vi "REPORT_AUDIT_get_data_results.vi"(6 "executed_SQL_statement_in":string, 8 "error_in":errorcluster, 11 "SQL_result":variant) -> (0 "error_out":errorcluster, 4 "executed_SQL_statement_out":string)   [LabVIEW 2020]
uses:
  FGV/SQL_connection/FGV_CLIENT_SQL_connection.ctl
  FGV/REPORTS_records_display/FGV_REPORTS_records_display.ctl
  _misc/AULocalize/SubVIs/Get Localized Phrase Compact Interface 0D.vi
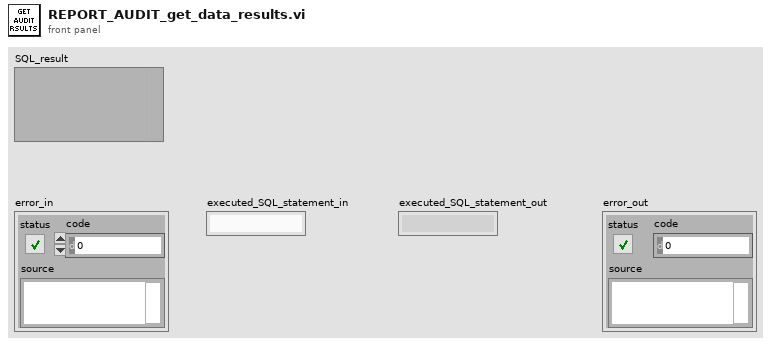
[diagram p1: front panel]
types:
  T1 = typedef "FGV_REPORTS_records_display.ctl" = enum16{"initialize", "GEAR_set_serial", "GEAR_set_header", "GEAR_set_operations", "GEAR_set_results", "GEAR_set_batches", "GEAR_get_serial", "GEAR_get_operation_IDs", "GEAR_toggle_results", "GEAR_show_all_results", "GEAR_hide_all_results", "GEAR_display", "GEAR_filter", "GEAR_restore", "GEAR_clear", "GEAR_get_all_info", "DATES_set_dates", "DATES_set_gears", "DATES_display", "DATES_filter", "DATES_first_page", "DATES_previous_page", "DATES_next_page", "DATES_last_page", "DATES_restore", "DATES_clear", "DATES_get_all_info", "PBATCH_set_batch_no", "PBATCH_set_gears", "PBATCH_display", "PBATCH_filter", "PBATCH_first_page", "PBATCH_previous_page", "PBATCH_next_page", "PBATCH_last_page", "PBATCH_restore", "PBATCH_clear", "PBATCH_get_all_info", "OPRTN_set_OP", "OPRTN_set_dates", "OPRTN_set_gears", "OPRTN_set_hidden_columns", "OPRTN_display", "OPRTN_filter", "OPRTN_filter_no_page_reset", "OPRTN_first_page", "OPRTN_previous_page", "OPRTN_next_page", "OPRTN_last_page", "OPRTN_restore", "OPRTN_clear", "OPRTN_get_all_info", "CFG_set_type", "CFG_set_dates", "CFG_set_records", "CFG_display", "CFG_filter", "CFG_first_page", "CFG_previous_page", "CFG_next_page", "CFG_last_page", "CFG_restore", "CFG_clear", "CFG_get_all_info", "AUDIT_set_dates", "AUDIT_set_records", "AUDIT_display", "AUDIT_filter", "AUDIT_first_page", "AUDIT_previous_page", "AUDIT_next_page", "AUDIT_last_page", "AUDIT_restore", "AUDIT_clear", "AUDIT_set_results", "AUDIT_get_all_info", "AUDIT_toggle_results", "AUDIT_show_all_results", "AUDIT_hide_all_results", "OKNOK_set_dates", "OKNOK_set_records", "OKNOK_display", "OKNOK_restore", "OKNOK_clear", "OKNOK_get_all_info", "REWORKS_set_dates", "REWORKS_set_from_to", "REWORKS_set_records", "REWORKS_display", "REWORKS_filter", "REWORKS_first_page", "REWORKS_previous_page", "REWORKS_next_page", "REWORKS_last_page", "REWORKS_restore", "REWORKS_clear", "REWORKS_get_all_info", "PACE_set_dates", "PACE_set_limits", "PACE_set_records", "PACE_display", "PACE_restore", "PACE_clear", "PACE_get_all_info", "CBATCH_set_code", "CBATCH_set_records", "CBATCH_display", "CBATCH_filter", "CBATCH_first_page", "CBATCH_previous_page", "CBATCH_next_page", "CBATCH_last_page", "CBATCH_restore", "CBATCH_clear", "CBATCH_get_all_info", "CMPNT_set_serial", "CMPNT_set_records", "CMPNT_display", "CMPNT_first_page", "CMPNT_previous_page", "CMPNT_next_page", "CMPNT_last_page", "CMPNT_restore", "CMPNT_clear", "CMPNT_get_all_info", "clear"}
  T2 = typedef "FGV_CLIENT_SQL_connection.ctl" = enum16{"initialize", "connect", "read_tables", "read_columns", "SELECT", "INSERT", "UPDATE", "DELETE", "EXEC + headers", "EXEC", "TRANSACTION", "connection_active?", "disconnect"}
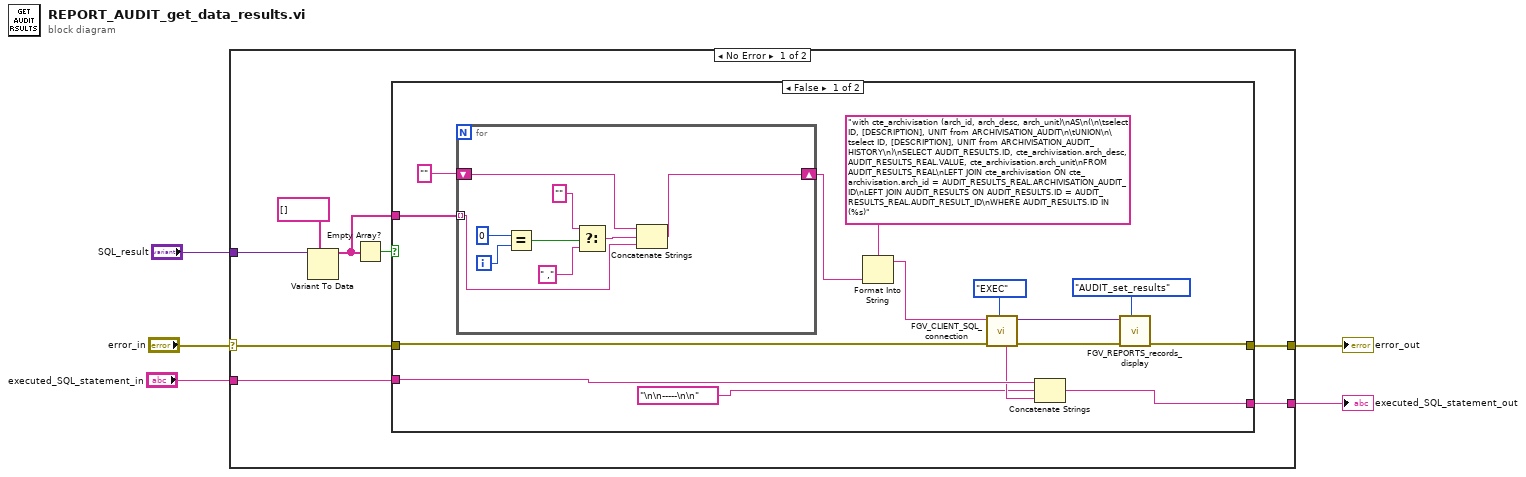
[diagram p0: block diagram]
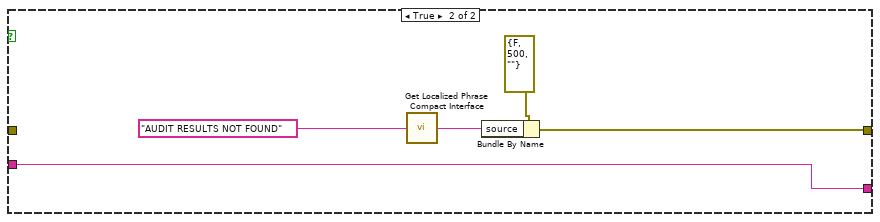
[diagram p2: hidden frame]
diagram:
  n1 = case shown="No Error" "error_in" {
    selector: "error_in" -> [w10 w44]
    tunnel: [w13 w43] -> w5
    tunnel: "executed_SQL_statement_in" -> [w12 w43]
    tunnel: [w11 w44] -> w3
    tunnel: "SQL_result" -> [w9 _]
    frame No Error {
      n2 = Variant To Data(type=string[] [], Variant=w9) -> (data=w7:string[])  [unwired: 1 in, 1 out]
      n3 = Empty Array?(array=w7) -> (empty?=w8:bool)
      n4 = case shown="False" w8 {
        tunnel: w10 -> [w28 _]
        tunnel: [w14 w38] -> w11
        tunnel: w12 -> [w21 w42]
        tunnel: [w18 w42] -> w13
        tunnel: w7 -> [w17 _]
        frame False {
          n5 = for {
            tunnel: w17 -> [w29] mode=indexing
            shift-right: [w30] -> w15
            shift-left: "" -> [w31]
            i -> [w35]
            n6 = Equal?(x=0, y=w35) -> (x = y?=w36:bool)
            n7 = Select(t="", s=w36, f=" ,") -> (s? t:f=w32:string)
            n8 = Concatenate Strings(w31, w32, w29) -> (w30:string)
          }
          n9 = Format Into String(format string="with cte_archivisation (arch_id, arch_desc, arch_unit)\nAS\n(\n\tselect ID, [DESCRIPTION], UNIT from ARCHIVISATION_AUDIT\n\tUNION\n\tselect ID, [DESCRIPTION], UNIT from ARCHIVISATION_AUDIT_HISTORY\n)\nSELECT AUDIT_RESULTS.ID, cte_archivisation.arch_desc, AUDIT_RESULTS_REAL.VALUE, cte_archivisation.arch_unit\nFROM AUDIT_RESULTS_REAL\nLEFT JOIN cte_archivisation ON cte_archivisation.arch_id = AUDIT_RESULTS_REAL.ARCHIVISATION_AUDIT_ID\nLEFT JOIN AUDIT_RESULTS ON AUDIT_RESULTS.ID = AUDIT_RESULTS_REAL.AUDIT_RESULT_ID\nWHERE AUDIT_RESULTS.ID IN (%s)", w15) -> (resulting string=w23:string)  [unwired: 2 in, 1 out]
          n10 = call "FGV_CLIENT_SQL_connection.vi"("options"=FGV_CLIENT_SQL_connection."EXEC", "error_in"=w28, "SQL_statement"=w23) -> ("error_out"=w25:errorcluster, "SQL_result"=w24:variant, "executed_SQL_statement"=w20:string)  [unwired: 4 in, 2 out]
          n11 = Concatenate Strings(w21, "\n\n-----\n\n" ("string"), w20) -> (w18:string)
          n12 = call "FGV_REPORTS_records_display.vi"("options"=FGV_REPORTS_records_display."AUDIT_set_results", "error_in"=w25, "input"=w24) -> ("error_out"=w14:errorcluster)  [unwired: 7 in, 1 out]
        }
        frame True {
          n13 = call-poly "Get Localized Phrase Compact Interface.vi"("Key"="AUDIT RESULTS NOT FOUND" ("source")) -> ("Translated Phrase"=w39:string)
          n14 = Bundle By Name(cluster=errorcluster {"status"=FALSE, "code"=500, "source"=""} ("error IO"), "source"=w39) -> (w38:errorcluster)
        }
      }
    }
    frame Error {
    }
  }
  "executed_SQL_statement_out" <- w5
  "error_out" <- w3
